vi "fgv_joystick_config.vi"(7 "cmd":T2, 8 "error in":errorcluster, 11 "Joystick cfg":T1={"Type"=enum."Logitech F710", "steer limit"={"min"=10.0, "max"=42.0, "scale"=0.0, "offset"=0.0}, "speed limit"={"min"=10.0, "max"=42.0, "pwm max"=0.0}, "ID"=0, "joystick max"=0.0}) -> (0 "error out":errorcluster, 3 "Joystick cfg out":T1={"Type"=enum."Logitech F710", "steer limit"={"min"=10.0, "max"=42.0, "scale"=0.0, "offset"=0.0}, "speed limit"={"min"=10.0, "max"=42.0, "pwm max"=0.0}, "ID"=0, "joystick max"=0.0})   [LabVIEW 2019]
uses:
  Ctrl/cmd_common.ctl
  Ctrl/joystick cfg.ctl
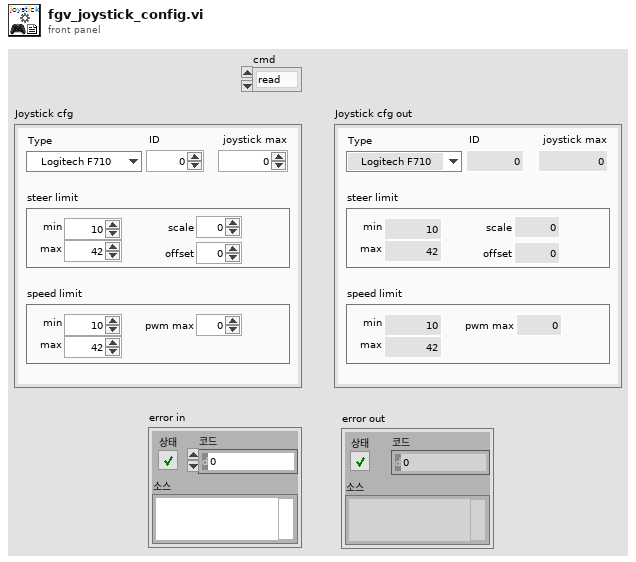
[diagram p1: front panel]
types:
  T1 = typedef "joystick cfg.ctl" = cluster{"Type":enum16{"Logitech F710", "Xbox"}, "steer limit":cluster{"min":dbl, "max":dbl, "scale":dbl, "offset":dbl}, "speed limit":cluster{"min":dbl, "max":dbl, "pwm max":dbl}, "ID":i32, "joystick max":dbl}
  T2 = typedef "cmd_common.ctl" = enum16{"read", "write"}
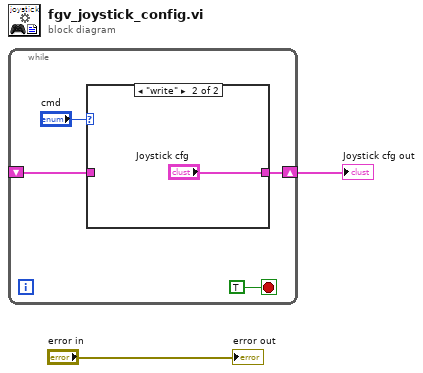
[diagram p0: block diagram]
diagram:
  n1 = while {
    shift-right: [w4] -> w2
    shift-left: _ -> [w3]
    stop <- TRUE stop-if-true
    n2 = case shown="\"write\"" "cmd" {
      tunnel: [w7 "Joystick cfg"] -> w4
      tunnel: w3 -> [w7 _]
      frame "read", Default {
      }
      frame "write" {
      }
    }
  }
  "Joystick cfg out" <- w2
  "error out" <- "error in"
